vi "Parse-Scan_Maze.vi"(9 "Scan Parameters":T1) -> (0 "Rows":T4[](array[typedef]), 1 "Barrier Coords":T2[](array[typedef]), 2 "Columns":T4[](array[typedef]))   [LabVIEW 2020]
doc: "<B>Description:</B> Recursively scan the maze pixel array to find where all the barriers are in the grid.\n\n<B>Date:</B> 06/2019\n<B>Author:</B> Luke Jarocki, Choose Movement Consulting, LLC"
uses:
  Controls/Scan_Values.ctl
  Controls/Parse-(X,Y).ctl
  Controls/TileColor.ctl
  Controls/Scan_Data.ctl
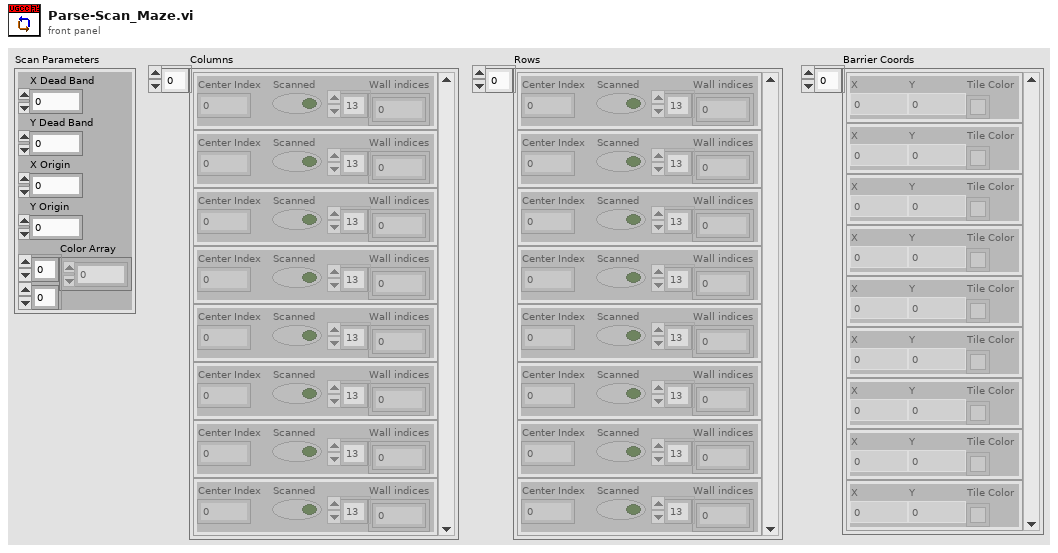
[diagram p1: front panel]
types:
  T1 = typedef "Scan_Data.ctl" = cluster{"X Dead Band":i32, "Y Dead Band":i32, "X Origin":i32, "Y Origin":i32, "Color Array":u32[][]}
  T2 = typedef "Parse-(X,Y).ctl" = cluster{"X":i32, "Y":i32, "Tile Color":T3}
  T3 = typedef "TileColor.ctl" = u16
  T4 = typedef "Scan_Values.ctl" = cluster{"Center Index":i32, "Scanned":bool, "Wall indices":i32[]}
  T5 = typedef "Wall Data.ctl" = cluster{"Wall indices":i32[], "Wall Center Index":i32, "Tile":T3}
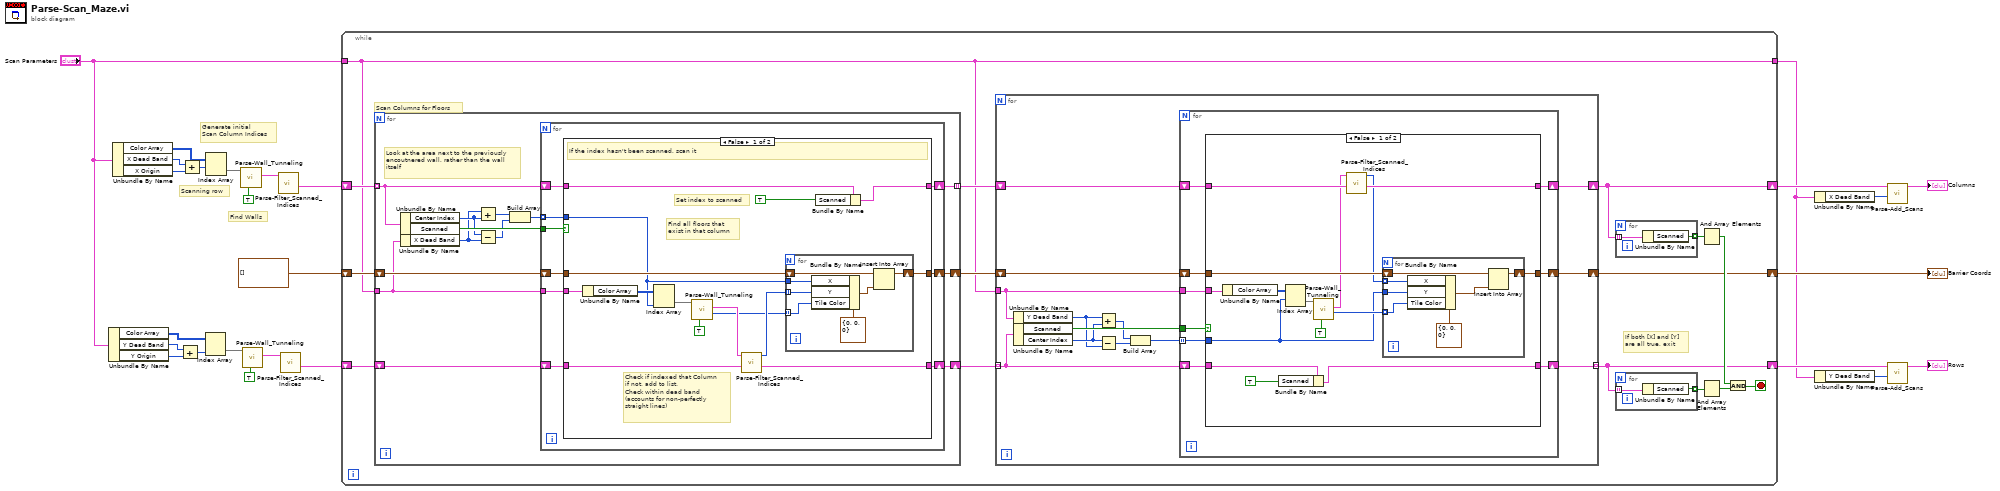
[diagram p0: block diagram]
diagram:
  # "Generate initial\nScan Column Indices"
  # "Find Walls"
  # "Scanning row"
  n1 = Unbundle By Name("Scan Parameters") -> ("Color Array"=w9:u32[][], "Y Dead Band"=w7:i32, "Y Origin"=w10:i32)
  n2 = Unbundle By Name("Scan Parameters") -> ("Color Array"=w19:u32[][], "X Dead Band"=w20:i32, "X Origin"=w21:i32)
  n3 = Add(x=w7, y=w10) -> (x+y=w11:i32)
  n4 = Add(x=w20, y=w21) -> (x+y=w24:i32)
  n5 = Index Array(array=w9, index (col)=w11) -> (element=w12:u32[])  [unwired: 1 in]
  n6 = Index Array(array=w19, index (row)=w24) -> (element=w26:u32[])  [unwired: 1 in]
  n7 = call "Parse-Wall_Tunneling.vi"("Tunnal All (F)"=TRUE, "Line to Parse"=w26) -> ("Wall Data"=w14:T5[])  [unwired: 6 in, 3 out]
  n8 = call "Parse-Wall_Tunneling.vi"("Tunnal All (F)"=TRUE, "Line to Parse"=w12) -> ("Wall Data"=w8:T5[])  [unwired: 6 in, 3 out]
  n9 = call "Parse-Filter_Scanned_Indices.vi"("Potential New Walls"=w14) -> ("Existing Indices Out"=w15:T4[])  [unwired: 9 in, 1 out]
  n10 = call "Parse-Filter_Scanned_Indices.vi"("Potential New Walls"=w8) -> ("Existing Indices Out"=w16:T4[])  [unwired: 9 in, 1 out]
  n11 = while {
    shift-right: [w33] -> w22
    shift-left: w15 -> [w41]
    shift-right: [w29] -> w17
    shift-left: w16 -> [w36]
    shift-right: [w30] -> w18
    shift-left: T2[] [] -> [w32]
    tunnel: "Scan Parameters" -> [w27]
    tunnel: [w27] -> w4
    stop <- w37 stop-if-true
    # "If both [X] and [Y]\nare all true, exit"
    # "Scan Columns for Floors"
    n12 = for {
      tunnel: w41 -> [w54] mode=indexing
      tunnel: [w53] -> w34 mode=indexing
      shift-right: [w50] -> w35
      shift-left: w36 -> [w51]
      shift-right: [w48] -> w31
      shift-left: w32 -> [w49]
      tunnel: w27 -> [w47]
      # "Look at the area next to the previously\nencoutnered wall, rather than the wall\nitself"
      n13 = Unbundle By Name(w54) -> ("Center Index"=w46:i32, "Scanned"=w52:bool)
      n14 = Unbundle By Name(w47) -> ("X Dead Band"=w45:i32)
      n15 = Add(x=w45, y=w46) -> (x+y=w44:i32)
      n16 = Subtract(x=w46, y=w45) -> (x-y=w43:i32)
      n17 = Build Array(w44, w43) -> (w42:i32[])
      n18 = for {
        tunnel: w47 -> [w56]
        tunnel: w42 -> [w55] mode=indexing
        shift-right: [w62] -> w53
        shift-left: w54 -> [w63]
        shift-right: [w59] -> w50
        shift-left: w51 -> [w60]
        shift-right: [w57] -> w48
        shift-left: w49 -> [w58]
        tunnel: w52 -> [w61]
        n19 = case shown="False" w61 {
          tunnel: w55 -> [w64 _]
          tunnel: w63 -> [w76 w88]
          tunnel: [w75 w88] -> w62
          tunnel: w60 -> [w73 w87]
          tunnel: [w72 w87] -> w59
          tunnel: w58 -> [w71 w86]
          tunnel: [w70 w86] -> w57
          tunnel: w56 -> [w69 _]
          frame False {
            # "Find all floors that\nexist in that column"
            # "Set index to scanned"
            # "Check if indexed that Column\nif not, add to list.\nCheck within dead band\n(accounts for non-perfectly\nstraight lines)"
            # "If the index hasn't been scanned, scan it"
            n20 = Unbundle By Name(w69) -> ("Color Array"=w68:u32[][])
            n21 = Index Array(array=w68, index (col)=w64) -> (element=w77:u32[])  [unwired: 1 in]
            n22 = call "Parse-Wall_Tunneling.vi"("Tunnal All (F)"=TRUE, "Line to Parse"=w77) -> ("Tile Type"=w65:T3[], "Wall Data"=w67:T5[])  [unwired: 6 in, 2 out]
            n23 = call "Parse-Filter_Scanned_Indices.vi"("Existing Indices"=w73, "Potential New Walls"=w67) -> ("Existing Indices Out"=w72:T4[], "New Wall Indices"=w66:i32[])  [unwired: 8 in]
            n24 = for {
              tunnel: w66 -> [w81] mode=indexing
              shift-right: [w84] -> w70
              shift-left: w71 -> [w85]
              tunnel: w64 -> [w80]
              tunnel: w65 -> [w79] mode=indexing
              n25 = Bundle By Name(cluster=T2 {"X"=0, "Y"=0, "Tile Color"=0}, "X"=w80, "Y"=w81, "Tile Color"=w79) -> (w82:T2)
              n26 = Insert Into Array(array=w85, new element=w82) -> (w84:T2[])  [unwired: 1 in]
            }
            n27 = Bundle By Name(cluster=w76, "Scanned"=TRUE) -> (w75:T4)
          }
          frame True {
            # "Index has been scanned, don't rescan"
          }
        }
      }
    }
    n28 = for {
      tunnel: w35 -> [w101] mode=indexing
      tunnel: [w100] -> w29 mode=indexing
      shift-right: [w98] -> w33
      shift-left: w34 -> [w99]
      shift-right: [w96] -> w30
      shift-left: w31 -> [w97]
      tunnel: w27 -> [w92]
      n29 = Unbundle By Name(w92) -> ("Y Dead Band"=w91:i32)
      n30 = Unbundle By Name(w101) -> ("Scanned"=w95:bool, "Center Index"=w93:i32)
      n31 = Add(x=w91, y=w93) -> (x+y=w94:i32)
      n32 = Subtract(x=w93, y=w91) -> (x-y=w90:i32)
      n33 = Build Array(w94, w90) -> (w89:i32[])
      n34 = for {
        tunnel: w92 -> [w104]
        tunnel: w89 -> [w102] mode=indexing
        shift-right: [w109] -> w100
        shift-left: w101 -> [w110]
        shift-right: [w107] -> w98
        shift-left: w99 -> [w108]
        shift-right: [w105] -> w96
        shift-left: w97 -> [w106]
        tunnel: w95 -> [w103]
        n35 = case shown="False" w103 {
          tunnel: w102 -> [w111 _]
          tunnel: w110 -> [w123 w135]
          tunnel: [w121 w135] -> w109
          tunnel: w108 -> [w120 w134]
          tunnel: [w119 w134] -> w107
          tunnel: w106 -> [w118 w133]
          tunnel: [w117 w133] -> w105
          tunnel: w104 -> [w116 _]
          frame False {
            n36 = Unbundle By Name(w116) -> ("Color Array"=w115:u32[][])
            n37 = Bundle By Name(cluster=w123, "Scanned"=TRUE ("Tunnal All (F)")) -> (w121:T4)
            n38 = Index Array(array=w115, index (row)=w111) -> (element=w125:u32[])  [unwired: 1 in]
            n39 = call "Parse-Wall_Tunneling.vi"("Tunnal All (F)"=TRUE, "Line to Parse"=w125) -> ("Tile Type"=w113:T3[], "Wall Data"=w114:T5[])  [unwired: 6 in, 2 out]
            n40 = call "Parse-Filter_Scanned_Indices.vi"("Existing Indices"=w120, "Potential New Walls"=w114) -> ("Existing Indices Out"=w119:T4[], "New Wall Indices"=w112:i32[])  [unwired: 8 in]
            n41 = for {
              shift-right: [w131] -> w117
              shift-left: w118 -> [w132]
              tunnel: w112 -> [w129] mode=indexing
              tunnel: w111 -> [w128]
              tunnel: w113 -> [w126] mode=indexing
              n42 = Bundle By Name(cluster=T2 {"X"=0, "Y"=0, "Tile Color"=0}, "X"=w129, "Y"=w128, "Tile Color"=w126) -> (w127:T2)
              n43 = Insert Into Array(array=w132, new element=w127) -> (w131:T2[])  [unwired: 1 in]
            }
          }
          frame True {
          }
        }
      }
    }
    n44 = for {
      tunnel: w33 -> [w139] mode=indexing
      tunnel: [w138] -> w40 mode=indexing
      n45 = Unbundle By Name(w139) -> ("Scanned"=w138:bool)
    }
    n46 = for {
      tunnel: w29 -> [w137] mode=indexing
      tunnel: [w136] -> w28 mode=indexing
      n47 = Unbundle By Name(w137) -> ("Scanned"=w136:bool)
    }
    n48 = And Array Elements(Boolean array=w40) -> (logical AND=w38:bool)
    n49 = And Array Elements(Boolean array=w28) -> (logical AND=w39:bool)
    n50 = And(x=w38, y=w39) -> (x .and. y?=w37:bool)
  }
  "Barrier Coords" <- w18
  n51 = Unbundle By Name(w4) -> ("X Dead Band"=w3:i32)
  n52 = Unbundle By Name(w4) -> ("Y Dead Band"=w2:i32)
  n53 = call "Parse-Add_Scans.vi"("Wall Thickness"=w3, "Existing Indices In"=w22) -> ("Indices With Scan"=→"Columns":T4[])  [unwired: 9 in]
  n54 = call "Parse-Add_Scans.vi"("Wall Thickness"=w2, "Existing Indices In"=w17) -> ("Indices With Scan"=→"Rows":T4[])  [unwired: 9 in]
